vi "PV ActiveLine - WatchdogControl.vi"(7 "W/R":bool, 8 "Fehler (Eingang)":errorcluster, 9 "Watchdog Set":u8(ring) items=["Manual error acknowledgement", "Automatic error acknowledgement (default)"], 11 "Referenz in":refnum<visa-resource-name>) -> (0 "Cluster (Ausgang)":errorcluster, 1 "Watchdog Get":u8(ring) items=["Manual error acknowledgement", "Automatic error acknowledgement (default)"], 3 "Referenz out":refnum<visa-resource-name>)   [LabVIEW 2013, in "PV ActiveLine.lvlib"]
doc: "WDT - Watchdog Control\n\nTransmit: WDT [,a]\nReceive: a\n\nWatchdog control, a =\n0 –> Manual error acknowledgement\n1 –> Automatic error acknowledgement (default)\n\nIf the watchdog has responded, the error is automatically acknowledged and cancelled after 2 s."
uses:
  <instrlib>/PV ActiveLine/PV ActiveLine.lvlib
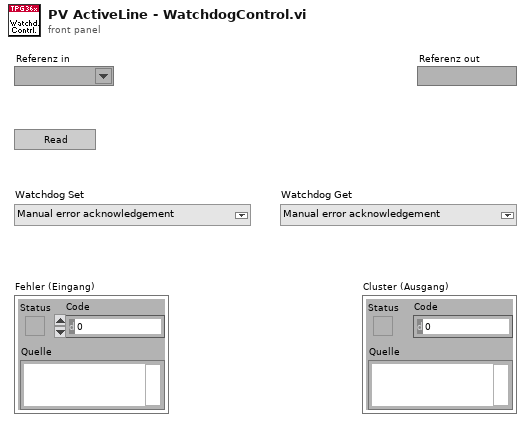
[diagram p1: front panel]
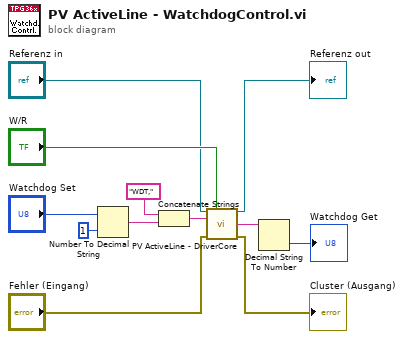
[diagram p0: block diagram]
diagram:
  n1 = Number To Decimal String(number="Watchdog Set", width (-)=i16 1) -> (decimal integer string=w7:string)
  n2 = Concatenate Strings("WDT,", w7) -> (w6:string)
  n3 = call <instrlib>:"PV ActiveLine - DriverCore.vi"("Referenz in"="Referenz in", "Write/Read"="W/R", "Command"=w6, "Fehler (Eingang)"="Fehler (Eingang)") -> ("Referenz out"=→"Referenz out":refnum<visa-resource-name>, "String Out"=w9:string, "Cluster (Ausgang)"=→"Cluster (Ausgang)":errorcluster)  [unwired: 9 in]
  n4 = Decimal String To Number(string=w9) -> (number=→"Watchdog Get":i32)  [unwired: 2 in, 1 out]
